vi "Load Config.vi"(8 "error in (no error)":errorcluster, 10 "Config_CSV_FilePath":path, 11 "MCLB_Template in":refnum<class "SCLB_Template.lvclass">) -> (0 "error out":errorcluster, 3 "MCLB_Template out":refnum<class "SCLB_Template.lvclass">)   [LabVIEW 2021, in "SCLB_Template.lvclass"]
uses:
  SCLB_Template.lvclass
  SCLB_Template.lvclass/SCLB_Template.ctl
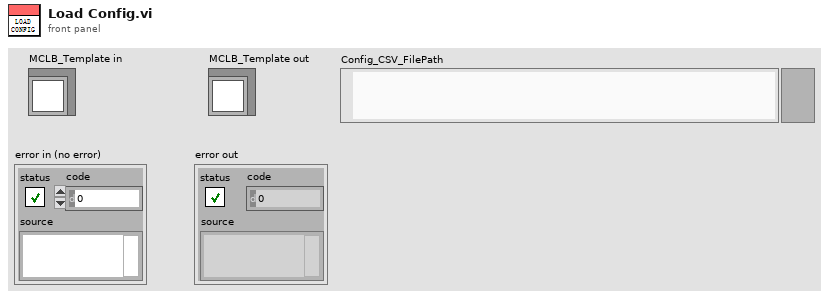
[diagram p1: front panel]
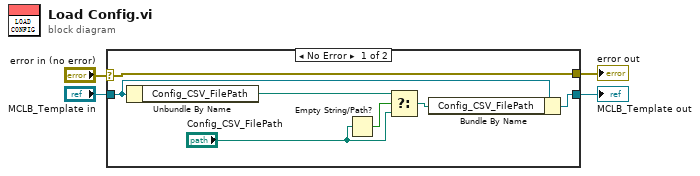
[diagram p0: block diagram]
diagram:
  n1 = case shown="No Error" "error in (no error)" {
    selector: "error in (no error)" -> [w11 w13]
    tunnel: [w11 w13] -> w3
    tunnel: [w6 w12] -> w1
    tunnel: "MCLB_Template in" -> [w7 w12]
    frame No Error {
      n2 = Unbundle By Name(w7) -> ("Config_CSV_FilePath"=w9:path)
      n3 = Empty String/Path?(string/path="Config_CSV_FilePath") -> (empty?=w10:bool)
      n4 = Select(t=w9, s=w10, f="Config_CSV_FilePath") -> (s? t:f=w5:path)
      n5 = Bundle By Name(cluster=w7, "Config_CSV_FilePath"=w5) -> (w6:refnum<class "SCLB_Template.lvclass">)
    }
    frame Error {
    }
  }
  "error out" <- w3
  "MCLB_Template out" <- w1
